vi "Edit Cell.vi"(8 "error in (no error)":errorcluster, 11 "DataGrid in":refnum<class "DataGrid.lvclass">) -> (0 "error out":errorcluster, 3 "DataGrid out":refnum<class "DataGrid.lvclass">)   [LabVIEW 2018, in "DataGrid.lvclass"]
uses:
  DataGrid.lvclass
  C:/Program Files (x86)/National Instruments/LabVIEW 2018/vi.lib/QSI/QControls/QControl Classes/MulticolumnListbox/MulticolumnListbox.lvclass
  DataGrid.lvclass/DataGrid.ctl
  <vilib>/MGI/Panel Manager/Panel/Panel/Window/Dialog/Dialog.lvclass
  C:/Program Files (x86)/National Instruments/LabVIEW 2018/vi.lib/MGI/Panel Manager/Panel/Panel/Panel.lvclass
  Read Current Edit Position.vi
  Read Configuration.vi
  <vilib>/QSI/DataGrid Configuration/DataGrid Config/DataGrid Config.lvclass
  <vilib>/QSI/DataGrid Configuration/Data Type Classes/Generic/Generic Data Type.lvclass
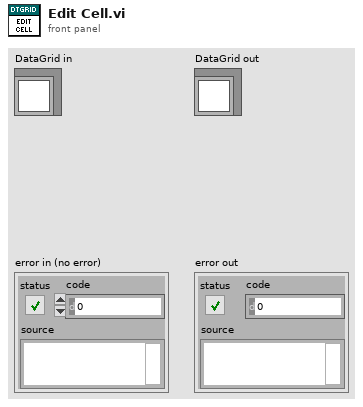
[diagram p1: front panel]
types:
  T1 = typedef "LVRowAndColumnTypeDef.ctl" = cluster{"Row":i32, "Column":i32}
  T2 = typedef "LVBoundsTypeDef.ctl" = cluster{"Width":u32, "Height":u32}
  T3 = typedef "LVPointTypeDef.ctl" = cluster{"Horizontal":i16, "Vertical":i16}
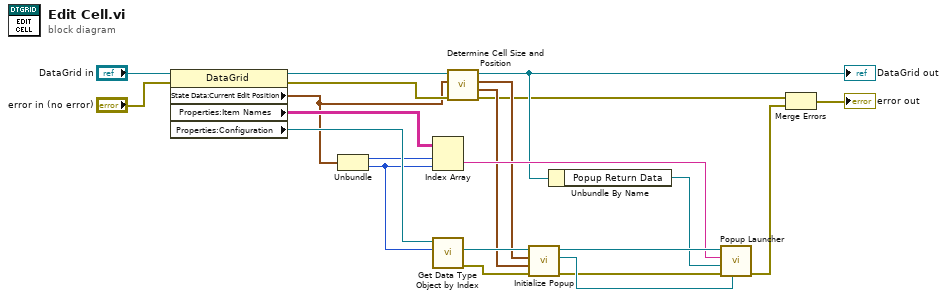
[diagram p0: block diagram]
diagram:
  n1 = property class="DataGrid"(reference="DataGrid in", error in="error in (no error)") -> (reference out=w7:refnum<class "DataGrid.lvclass">, error out=w5:errorcluster, "State Data:Current Edit Position"=w4:T1, "Properties:Item Names"=w21:string[][], "Properties:Configuration"=w22:refnum<class "DataGrid Config.lvclass">)
  n2 = Unbundle(w4) -> ("Row"=w10:i32, "Column"=w12:i32)
  n3 = Index Array(array=w21, index (row)=w10, index (col)=w12) -> (element=w11:string)
  n4 = call <vilib>:"Get Data Type Object by Index.vi"("Index"=w12, "DataGrid Config in"=w22) -> ("error out"=w18:errorcluster, "Data Type Object"=w14:refnum<class "Generic Data Type.lvclass">)  [unwired: 7 in, 1 out]
  n5 = call "Determine Cell Size and Position.vi"("error in (no error)"=w5, "Cell Position"=w4, "DataGrid in"=w7) -> ("error out"=w1:errorcluster, "Properties:Active Cell Cell Size"=w2:T2, "ScreenCoords"=w3:T3, "DataGrid out"=w6:refnum<class "DataGrid.lvclass">)  [unwired: 5 in]
  "DataGrid out" <- w6
  n6 = call-dynamic "Initialize Popup.vi"("error in (no error)"=w18, "Size"=w2, "Screen Coordinates"=w3, "Generic Data Type in"=w14) -> ("error out"=w16:errorcluster, "Dialog"=w17:refnum<class "Dialog.lvclass">, "Generic Data Type out"=w15:refnum<class "Generic Data Type.lvclass">)  [unwired: 5 in]
  n7 = Unbundle By Name(w6) -> ("Popup Return Data"=w13:refnum<user-event>)
  n8 = call <vilib>:"Popup Launcher.vi"("Panel"=w17, "error in (no error)"=w16, "Popup Return Data"=w13, "String in"=w11, "Generic Data Type in"=w15) -> ("error out"=w20:errorcluster)  [unwired: 5 in, 1 out]
  n9 = Merge Errors(w1, w20) -> (→"error out":errorcluster)
